vi "TMP36SubVI.vi"(1 "Raw Input (V)":dbl) -> (0 "Temperature (C)":dbl)   [LabVIEW 2017]
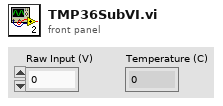
[diagram p1: front panel]
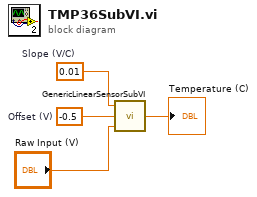
[diagram p0: block diagram]
diagram:
  w2 = -0.5  # Offset (V)
  w3 = 0.01  # Slope (V/C)
  n1 = call "GenericLinearSensorSubVI.vi"("Raw Input"="Raw Input (V)", "Offset"=w2, "Slope"=w3) -> ("Scaled Output"=→"Temperature (C)":dbl)
